vi "discardCommandsWithBadChecksum.vi"(10 "multi-line string":string) -> (2 "outputstring":string)   [LabVIEW 2013, in "Utilities.lvlib"]
uses:
  classes/Devices/emTestCWS500N/EMTestCWS500N.lvclass
  lib/Utilities.lvlib
panel:
  out "outputstring 2":string
  out "match substring":string
  out "offset past match":i32
  out "output":string
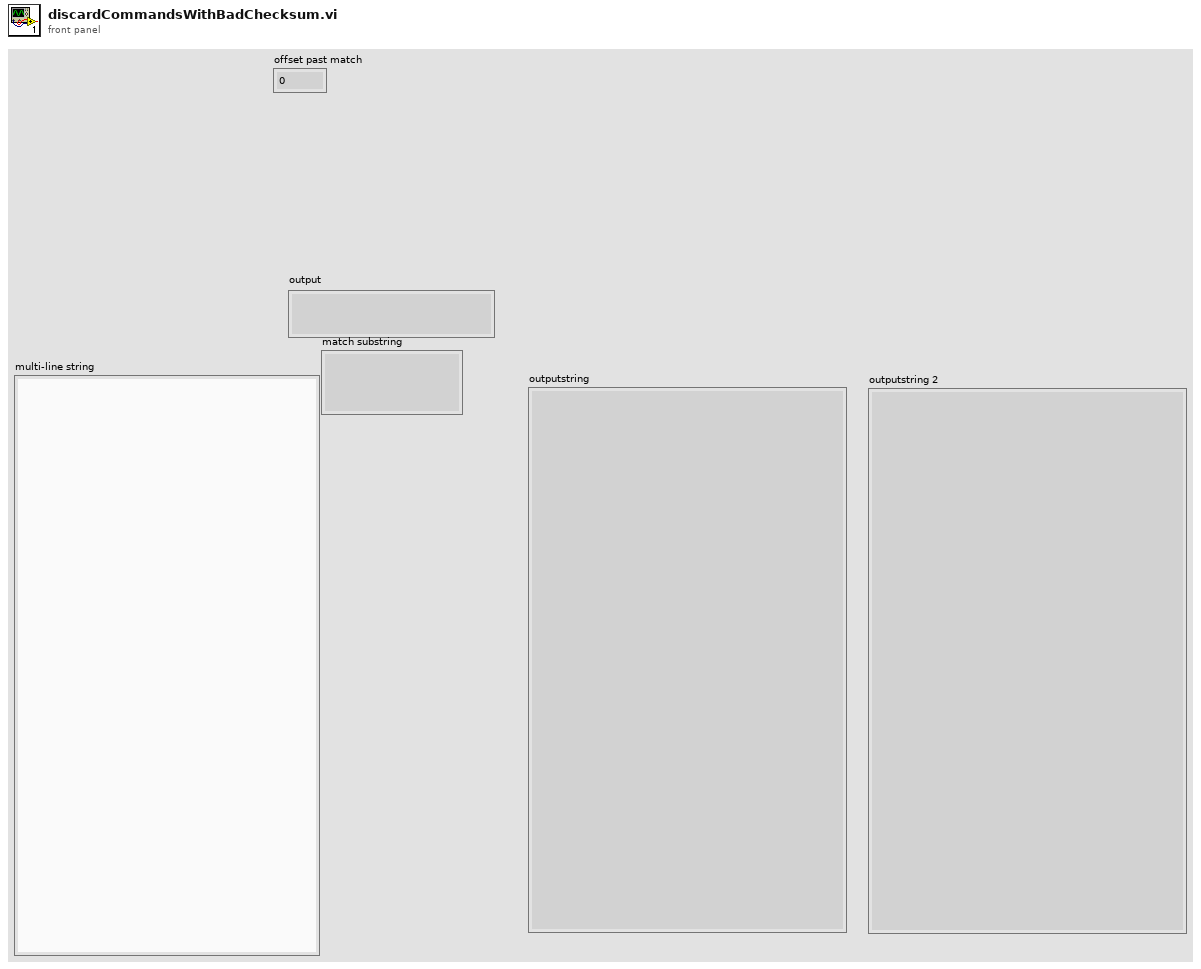
[diagram p1: front panel]
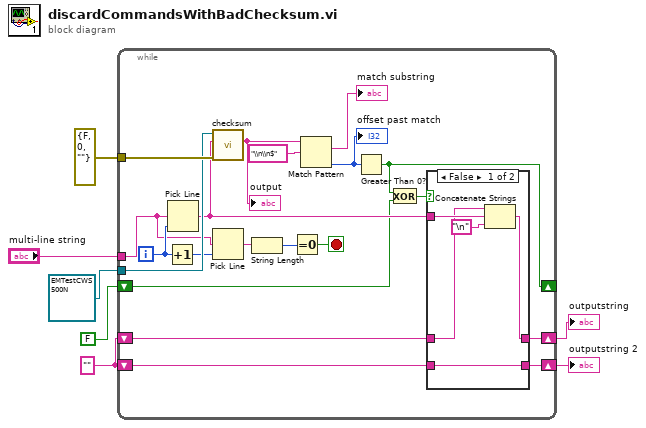
[diagram p0: block diagram]
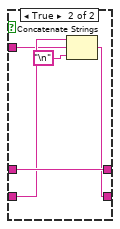
[diagram p2: hidden frame]
diagram:
  w2 = ""
  n1 = while {
    tunnel: errorcluster {"status"=FALSE, "code"=0, "source"=""} ("error out") -> [w27]
    tunnel: refnum<class "EMTestCWS500N.lvclass"> refnum ("EMTestCWS500N.lvclass") -> [w26]
    tunnel: "multi-line string" -> [w20]
    shift-right: [w14] -> w4
    shift-left: w2 -> [w15]
    shift-right: [w13] -> w3
    shift-left: w2 -> [w12]
    shift-right: [w9] -> _
    shift-left: FALSE -> [w10]
    i -> [w24]
    stop <- w21 stop-if-true
    n2 = Increment(x=w24) -> (x+1=w25:i32)
    n3 = Pick Line(multi-line string=w20, line index=w24) -> (output string=w11:string)  [unwired: 1 in]
    n4 = call-dynamic "checksum.vi"("error in (no error)"=w27, "input"=w11, "EMTestCWS500N in"=w26) -> ("output"=w16:string)  [unwired: 6 in, 2 out]
    "output" <- w16
    n5 = Pick Line(multi-line string=w20, line index=w25) -> (output string=w23:string)  [unwired: 1 in]
    n6 = String Length(string=w23) -> (length=w22:i32)
    n7 = Equal To 0?(x=w22) -> (x = 0?=w21:bool)
    n8 = Match Pattern(string=w16, regular expression="\\n\\n$") -> (match substring=→"match substring":string, offset past match=w17:i32)  [unwired: 1 in, 2 out]
    "offset past match" <- w17
    n9 = Greater Than 0?(x=w17) -> (x > 0?=w9:bool)
    n10 = Exclusive Or(1:w10, 2:w9) -> (0:w8:bool)
    n11 = case shown="False" w8 {
      tunnel: w11 -> [w32 w34]
      tunnel: w15 -> [w31 w37]
      tunnel: [w30 w37] -> w14
      tunnel: [w29 w35] -> w13
      tunnel: w12 -> [w29 w36]
      frame False {
        n12 = Concatenate Strings(w31, w32, "\n") -> (w30:string)
      }
      frame True {
        n13 = Concatenate Strings(w36, w34, "\n") -> (w35:string)
      }
    }
  }
  "outputstring" <- w4
  "outputstring 2" <- w3
